vi "Execute.vi"(8 "error in (no error)":errorcluster, 10 "Abstract Consumer in":refnum<class "Abstract Consumer.lvclass">, 11 "Consumer Name Request Message in":refnum<class "Consumer Name Request Message.lvclass">) -> (0 "error out":errorcluster, 1 "Abstract Response out":refnum<class "Abstract Response Message.lvclass">, 2 "Abstract Consumer out":refnum<class "Abstract Consumer.lvclass">, 3 "Consumer Name Request Message out":refnum<class "Consumer Name Request Message.lvclass">, 4 "Stop?":bool)   [LabVIEW 2017, in "Consumer Name Request Message.lvclass"]
uses:
  Consumer Name Request Message.lvclass
  Consumer/Abstract Consumer/Abstract Consumer.lvclass
  Message/Abstract Response Message/Abstract Response Message.lvclass
  Consumers/Test Consumer/Test Consumer.lvclass
  Consumer Name Response Message/Consumer Name Response Message.lvclass
  C:/github/niveristand-custom-device-message-library/Source/Message/Abstract Response Message/Abstract Response Message.lvclass
  Message List Action.ctl
  Consumers/Test Consumer/Test Consumer.lvclass/Test Consumer.ctl
  Consumer Name Response Message/Consumer Name Response Message.lvclass/Consumer Name Response Message.ctl
  Consumers/Test Consumer/Read Consumer Name.vi
  Consumer Name Response Message/Write Consumer Name.vi
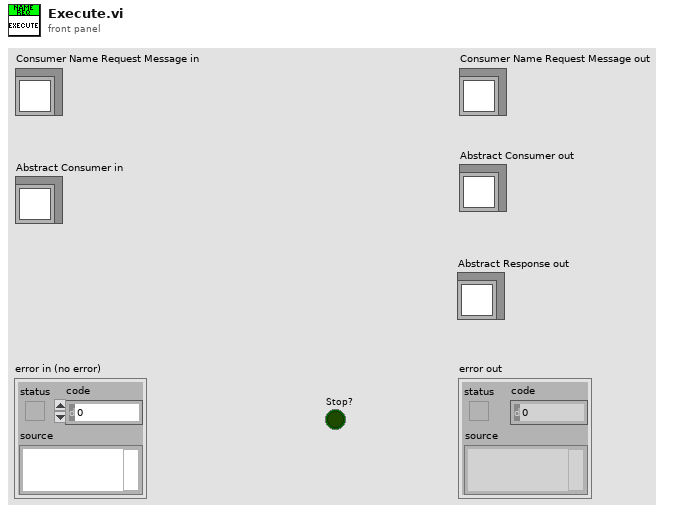
[diagram p1: front panel]
types:
  T1 = typedef "Message List Action.ctl" = enum16{"Get", "Add", "Reset"}
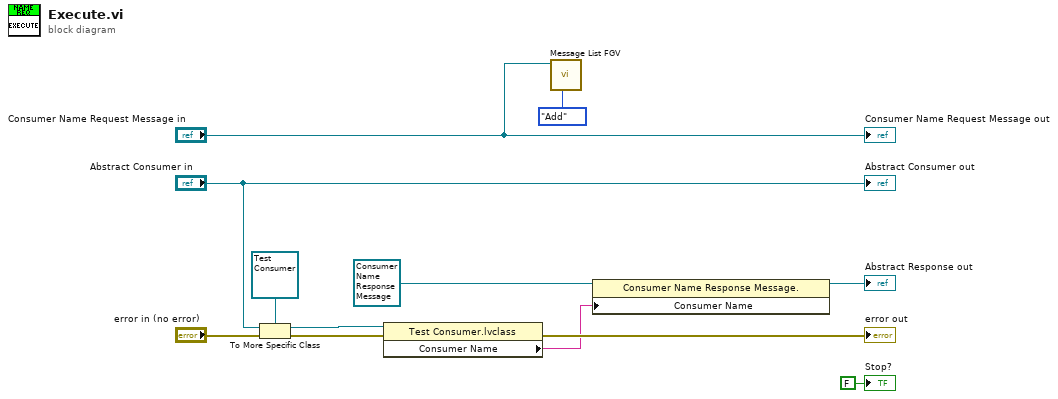
[diagram p0: block diagram]
diagram:
  n1 = To More Specific Class(target class=refnum<class "Test Consumer.lvclass"> refnum ("Reflected Name Consumer.lvclass"), reference="Abstract Consumer in", error in="error in (no error)") -> (specific class reference=w8:refnum<class "Test Consumer.lvclass">, error out=w9:errorcluster)
  n2 = property class="Test Consumer.lvclass"(reference=w8, error in=w9) -> (error out=→"error out":errorcluster, "Consumer Name"=w5:string)  [unwired: 1 out]
  n3 = call "Message List FGV.vi"("Action (Get)"=Message_List_Action."Add", "Message Object"="Consumer Name Request Message in") -> ()  [unwired: 8 in, 2 out]
  n4 = property class="Consumer Name Response Message."(reference=refnum<class "Consumer Name Response Message.lvclass"> refnum ("Consumer Name Response Message.lvclass"), "Consumer Name"=w5) -> (reference out=→"Abstract Response out":refnum<class "Consumer Name Response Message.lvclass">)  [unwired: 1 in, 1 out]
  "Consumer Name Request Message out" <- "Consumer Name Request Message in"
  "Abstract Consumer out" <- "Abstract Consumer in"
  "Stop?" <- FALSE ("Stop?")
